vi "Simulated Thermocouple GUID Lookup.vi"() -> ()   [LabVIEW 2011, in "Simulated Thermocouple Custom Device.lvlib"]
doc: "Use this Global VI to access the GUIDs assigned to the page resources of the Custom Device."
uses:
  Simulated Thermocouple Custom Device.lvlib
panel:
  in  "TC Calibration Config":string="3027efba-c0b5-45a3-8ca2-970824ba31f4"
  in  "TC Channel Config":string="b04bcaf6-e16e-4f2b-a421-09dcc5771ba7"
  in  "CO Channel Config":string="3b7fd3f7-897f-48c1-a62a-0ee2e9a994a1"
  in  "VO Channel Config":string="31dee1d3-8e49-4944-be8e-483cab571167"
  in  "Simulated Thermocouples":string="58e2782a-ff74-4e3c-99e5-d50d5b53a861"
  in  "Current Outputs":string="4997e311-51b7-4029-a044-e2490122e7ac"
  in  "Voltage Outputs":string="a01dde1d-2391-43a9-8263-697254600c9d"
  in  "Custom Device":string="32ef703f-981c-427b-acef-84d810e0c668"
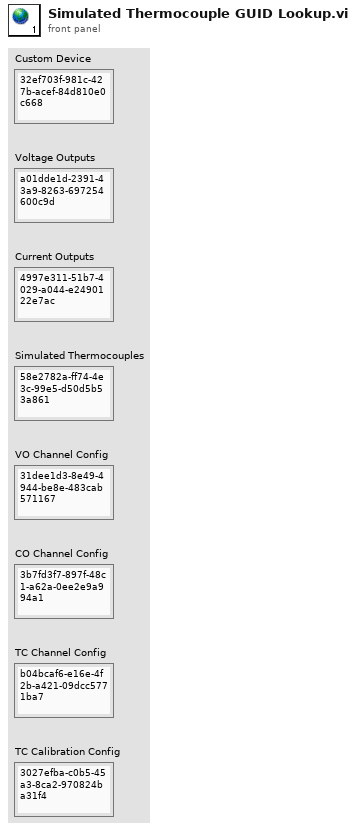
[diagram p1: front panel]
diagram:
